vi "translateObj.vi"(8 "POI_proj_Offset (0,0,0)":cluster{"X":dbl, "Y":dbl, "Z":dbl}, 9 "vector":cluster{"X":dbl, "Y":dbl, "Z":dbl}, 10 "Type":string, 11 "Scene: Object":refnum<vi>) -> (0 "error out":errorcluster, 3 "dub Scene Object":refnum<vi>)   [LabVIEW 2015]
uses:
  <vilib>/picture/3D Picture Control/NI_3D Picture Control.lvlib
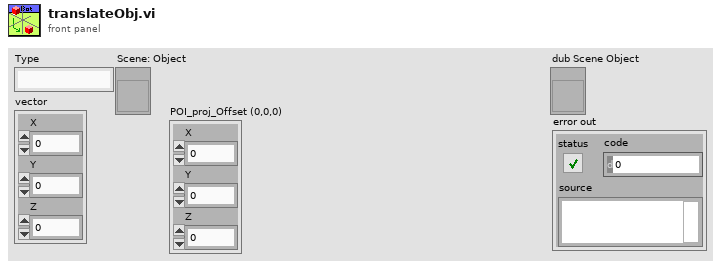
[diagram p1: front panel]
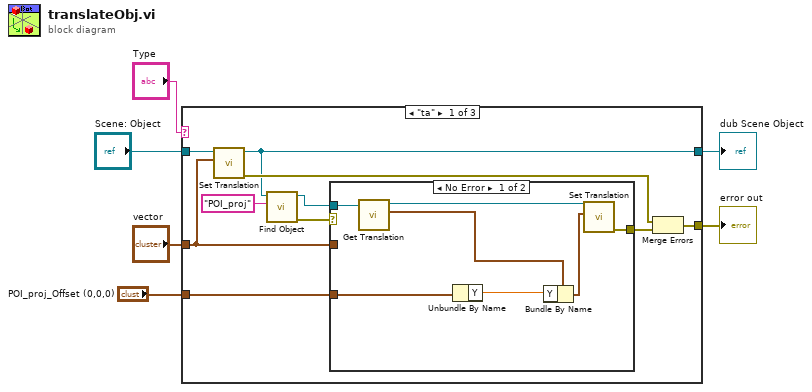
[diagram p0: block diagram]
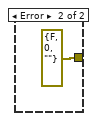
[diagram p2: hidden frame]
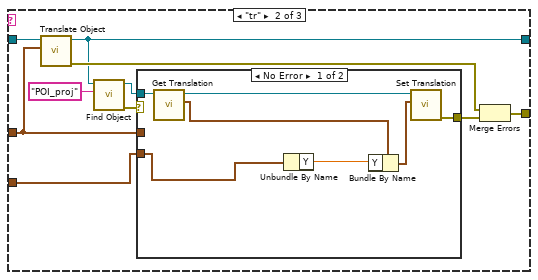
[diagram p3: hidden frame]
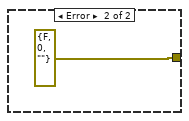
[diagram p4: hidden frame]
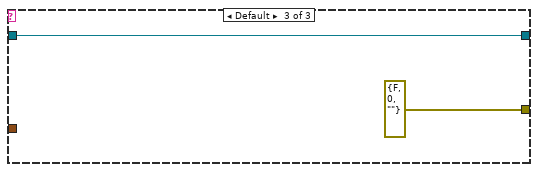
[diagram p5: hidden frame]
diagram:
  n1 = case shown="\"ta\"" "Type" {
    tunnel: "vector" -> [w12 w30 _]
    tunnel: "Scene: Object" -> [w13 w31 w44]
    tunnel: [w7 w25 w44] -> w3
    tunnel: [w9 w27 errorcluster {"status"=FALSE, "code"=0, "source"=""} ("error out")] -> w2
    tunnel: "POI_proj_Offset (0,0,0)" -> [w8 w26 _]
    frame "ta" {
      n2 = call <vilib>:"Set Translation.vi"("Translation"=w12, "Scene Object"=w13) -> ("error out"=w10:errorcluster, "Translated Object"=w7:refnum<vi>)  [unwired: 8 in]
      n3 = call <vilib>:"Find Object.vi"("Object Name"="POI_proj", "Scene Refnum"=w7) -> ("error out"=w15:errorcluster, "Object Refnum"=w14:refnum<vi>)  [unwired: 8 in]
      n4 = case shown="No Error" w15 {
        tunnel: w14 -> [w21 _]
        tunnel: w12 -> [_ _]
        tunnel: [w22 errorcluster {"status"=FALSE, "code"=0, "source"=""} ("error out")] -> w11
        tunnel: w8 -> [w17 _]
        frame No Error {
          n5 = call <vilib>:"Get Translation.vi"("Scene Object"=w21) -> ("Transformation:Get Translation"=w19:cluster{"X":sgl, "Y":sgl, "Z":sgl}, "Scene Object"=w20:refnum<vi>)  [unwired: 8 in, 1 out]
          n6 = Unbundle By Name(w17) -> ("Y"=w18:dbl)
          n7 = Bundle By Name(cluster=w19, "Y"=w18) -> (w23:cluster{"X":sgl, "Y":sgl, "Z":sgl})
          n8 = call <vilib>:"Set Translation.vi"("Translation"=w23, "Scene Object"=w20) -> ("error out"=w22:errorcluster)  [unwired: 8 in, 1 out]
        }
        frame Error {
        }
      }
      n9 = Merge Errors(w10, w11) -> (w9:errorcluster)
    }
    frame "tr" {
      n10 = call <vilib>:"Translate Object.vi"("Translation"=w30, "Scene.Object In"=w31) -> ("error out"=w28:errorcluster, "Scene.Object Out"=w25:refnum<vi>)  [unwired: 8 in]
      n11 = call <vilib>:"Find Object.vi"("Object Name"="POI_proj", "Scene Refnum"=w25) -> ("error out"=w33:errorcluster, "Object Refnum"=w32:refnum<vi>)  [unwired: 8 in]
      n12 = case shown="No Error" w33 {
        tunnel: w32 -> [w39 _]
        tunnel: w30 -> [_ _]
        tunnel: [w40 errorcluster {"status"=FALSE, "code"=0, "source"=""} ("error out")] -> w29
        tunnel: w26 -> [w35 _]
        frame No Error {
          n13 = call <vilib>:"Get Translation.vi"("Scene Object"=w39) -> ("Transformation:Get Translation"=w37:cluster{"X":sgl, "Y":sgl, "Z":sgl}, "Scene Object"=w38:refnum<vi>)  [unwired: 8 in, 1 out]
          n14 = Unbundle By Name(w35) -> ("Y"=w36:dbl)
          n15 = Bundle By Name(cluster=w37, "Y"=w36) -> (w41:cluster{"X":sgl, "Y":sgl, "Z":sgl})
          n16 = call <vilib>:"Set Translation.vi"("Translation"=w41, "Scene Object"=w38) -> ("error out"=w40:errorcluster)  [unwired: 8 in, 1 out]
        }
        frame Error {
        }
      }
      n17 = Merge Errors(w28, w29) -> (w27:errorcluster)
    }
    frame Default {
    }
  }
  "dub Scene Object" <- w3
  "error out" <- w2
